vi "Gross Weight.vi"(8 "error in (no error)":errorcluster, 11 "Instrument.LN2 in":refnum<class "Instrument.LN2.lvclass">) -> (0 "error out":errorcluster, 2 "Get Weight":dbl, 3 "Instrument.LN2 out":refnum<class "Instrument.LN2.lvclass">)   [LabVIEW 2019, in "Instrument.LN2.lvclass"]
uses:
  Instrument.LN2.lvclass
  Instrument.LN2.lvclass/Instrument.LN2.ctl
  <vilib>/regexp/Match Regular Expression.xnode
panel:
  out "before match":string
  out "after match":string
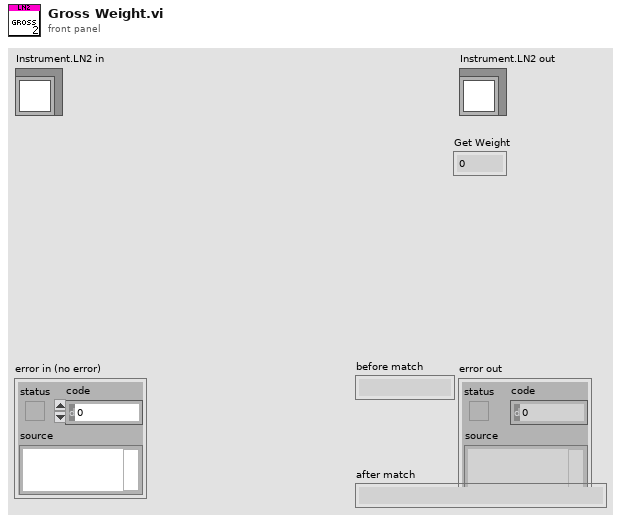
[diagram p1: front panel]
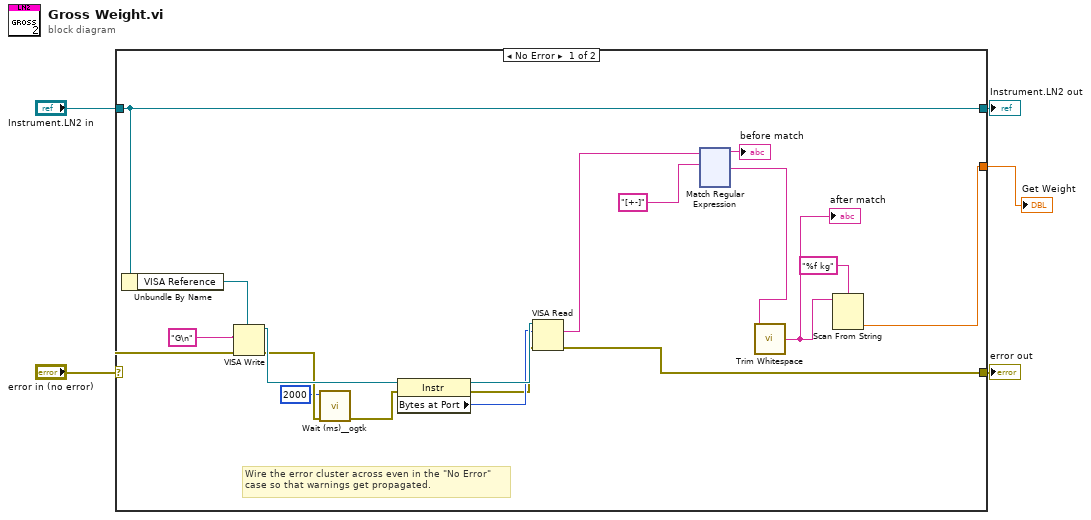
[diagram p0: block diagram]
diagram:
  n1 = case shown="No Error" "error in (no error)" {
    selector: "error in (no error)" -> [w21 w140]
    tunnel: [w20 w140] -> w4
    tunnel: [w24 w139] -> w2
    tunnel: "Instrument.LN2 in" -> [w24 w139]
    tunnel: [w13 _] -> w1
    frame No Error {
      # "Wire the error cluster across even in the \"No Error\"\ncase so that warnings get propagated."
      n2 = Unbundle By Name(w24) -> ("VISA Reference"=w23:refnum<visa-resource-name>)
      n3 = VISA Write(VISA resource name=w23, write buffer="G\n", error in (no error)=w21) -> (VISA resource name out=w12:refnum<visa-resource-name>, error out=w9:errorcluster)  [unwired: 1 out]
      n4 = call <userlib>:"Wait (ms)__ogtk.vi"("error in (no error)"=w9, "milliseconds to wait"=u32 2000) -> ("error out"=w7:errorcluster)  [unwired: 8 in, 1 out]
      n5 = property on="Property Node" class="Instr"(reference=w12, error in=w7) -> (reference out=w11:refnum<visa-resource-name>, error out=w6:errorcluster, "Bytes at Port"=w10:u32)
      n6 = VISA Read(VISA resource name=w11, byte count=w10, error in (no error)=w6) -> (read buffer=w14:string, error out=w20:errorcluster)  [unwired: 2 out]
      n7 = xnode "Match Regular Expression"("input string"=w14, "regular expression"="[+-]" ("format string")) -> ("before match"=→"before match":string, "after match"=w16:string)  [unwired: 4 in, 3 out]
      n8 = call <vilib>:"Trim Whitespace.vi"("string"=w16) -> ("trimmed string"=w15:string)  [unwired: 1 in]
      "after match" <- w15
      n9 = Scan From String(format string="%f kg", input string=w15) -> (output 1=w13:dbl)  [unwired: 3 in, 3 out]
    }
    frame Error {
    }
  }
  "error out" <- w4
  "Instrument.LN2 out" <- w2
  "Get Weight" <- w1
